vi "Instrument jsObject Array.vi"(8 "error in (no error)":errorcluster, 9 "Instruments (empty)":T1[](array[typedef]), 10 "Instruments jsObject Array Name (\"INSTRUMENTS\")":string="INSTRUMENTS", 11 "Previous String (\"\")":string) -> (0 "error out":errorcluster, 2 "Instruments jsObject Array":string, 3 "Instrument Definition":string)   [LabVIEW 2011]
uses:
  Instrument Record.ctl
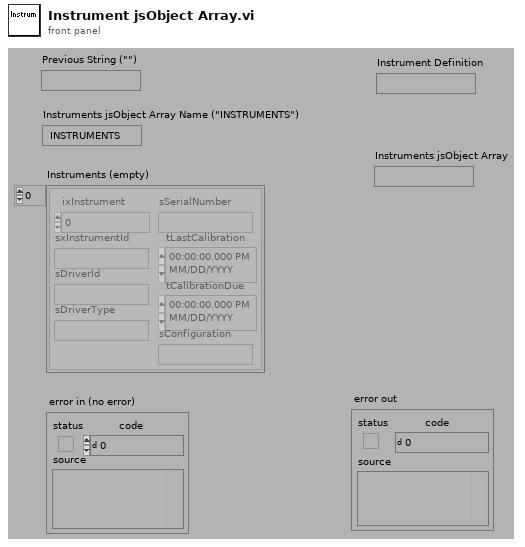
[diagram p1: front panel]
types:
  T1 = typedef "Instrument Record.ctl" = cluster{"ixInstrument":i32, "sxInstrumentId":string, "sDriverId":string, "sDriverType":string, "sSerialNumber":string, "tLastCalibration":timestamp, "tCalibrationDue":timestamp, "sConfiguration":string}
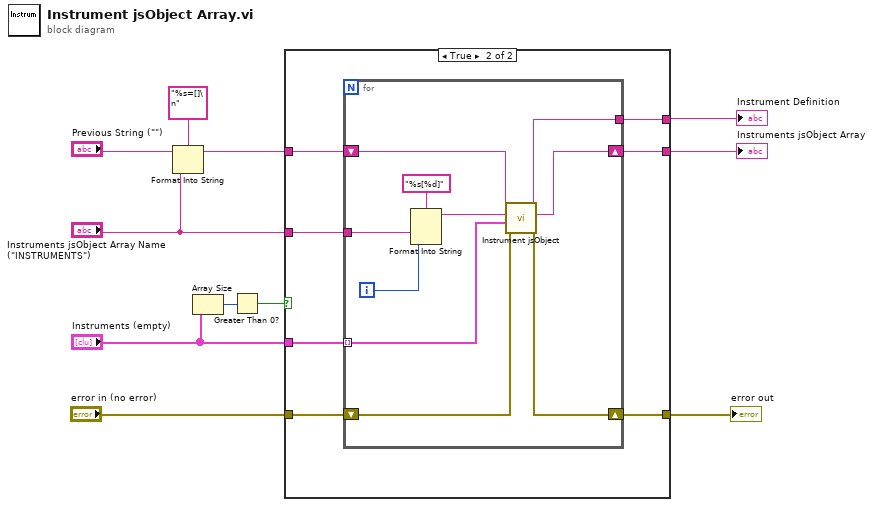
[diagram p0: block diagram]
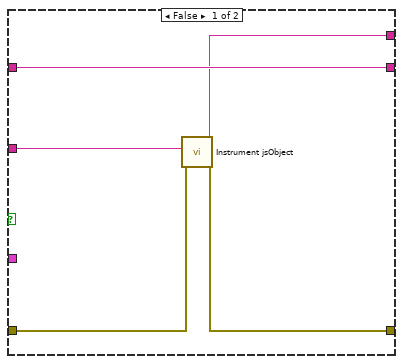
[diagram p2: hidden frame]
diagram:
  n1 = Format Into String(format string="%s=[]\n", initial string="Previous String (\"\")", "Instruments jsObject Array Name (\"INSTRUMENTS\")") -> (resulting string=w10:string)  [unwired: 1 in, 1 out]
  n2 = Array Size(array="Instruments (empty)") -> (size(s)=w9:i32)
  n3 = Greater Than 0?(x=w9) -> (x > 0?=w8:bool)
  n4 = case shown="True" w8 {
    tunnel: w10 -> [w16 w23]
    tunnel: "error in (no error)" -> [w15 w22]
    tunnel: [w16 w21] -> w3
    tunnel: [w14 w20] -> w2
    tunnel: "Instruments jsObject Array Name (\"INSTRUMENTS\")" -> [w13 w19]
    tunnel: [w12 w18] -> w1
    tunnel: "Instruments (empty)" -> [_ w17]
    frame False {
      n5 = call "Instrument jsObject.vi"("error in (no error)"=w15, "Instrument Object Name (\"\")"=w13) -> ("error out"=w14:errorcluster, "Instrument Definition"=w12:string)  [unwired: 2 in, 6 out]
    }
    frame True {
      n6 = for {
        tunnel: w17 -> [w27] mode=indexing
        shift-right: [w25] -> w21
        shift-left: w23 -> [w29]
        shift-right: [w24] -> w20
        shift-left: w22 -> [w26]
        tunnel: w19 -> [w32]
        tunnel: [w30] -> w18
        i -> [w31]
        n7 = Format Into String(format string="%s[%d]", w32, w31) -> (resulting string=w28:string)  [unwired: 2 in, 1 out]
        n8 = call "Instrument jsObject.vi"("error in (no error)"=w26, "Instrument Record (empty)"=w27, "Instrument Object Name (\"\")"=w28, "Previous String (\"\")"=w29) -> ("error out"=w24:errorcluster, "Instrument jsObject"=w25:string, "Instrument Definition"=w30:string)  [unwired: 5 out]
      }
    }
  }
  "Instruments jsObject Array" <- w3
  "error out" <- w2
  "Instrument Definition" <- w1
